vi "Update_FFID_Bkgnd_info.vi"(1 "Specific Bkgnd Meas?":bool, 2 "c^2 (ppm^2)":dbl[](array[numeric]), 3 "C (ppm)":dbl[](array[numeric])) -> ()   [LabVIEW 2010]
uses:
  Globals/Meas_global.vi
  Globals/Plug_in_data_global.vi
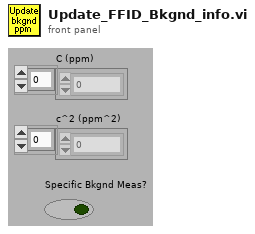
[diagram p1: front panel]
types:
  T1 = typedef "Analysis_info_cluster.ctl" = cluster{"Colour":u32, "Inst type":T2, "Inst name":string, "Symbol":string, "Code name":string, "Extra Info":string, "Inst Array":T3, "Index":i32, "Voltage Index":i32, "Extra Titles":string[], "Extra Values":string[]}
  T2 = typedef "Inst_type.ctl" = enum16{"Propeller anemometer", "Raw voltage", "Pressure Transducer", "Pitot-static tube", "Preston tube", "Hot wire", "Cross wire 1", "Cross wire 2", "Generic Linear", "Generic Polynomial", "Generic BackPoly", "Fast FID", "Thermocouple", "Cold wire", "Pulsed Wire", "LDA Vel", "LDA Tran time", "LDA Arr time"}
  T3 = typedef "Instrument_Array.ctl" = enum16{"PWA", "LDA", "Analogue"}
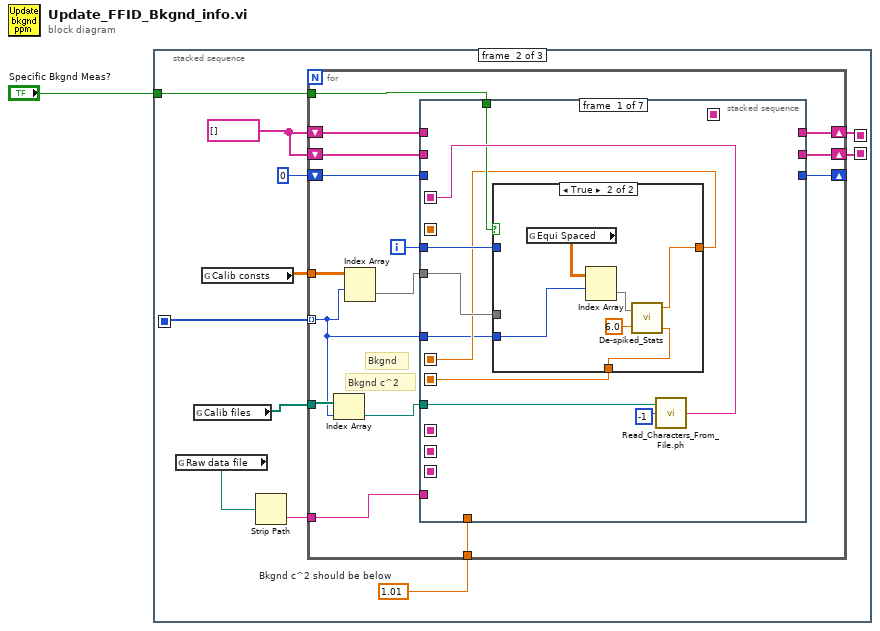
[diagram p0: block diagram]
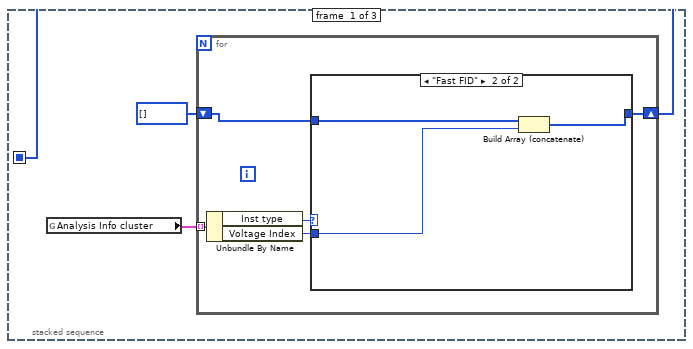
[diagram p2: hidden frame]
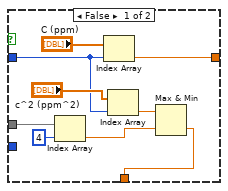
[diagram p4: hidden frame]
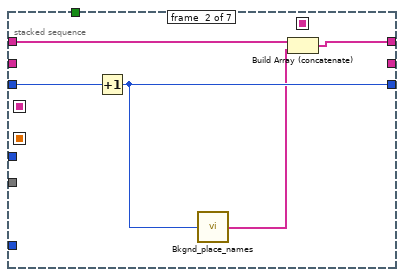
[diagram p5: hidden frame]
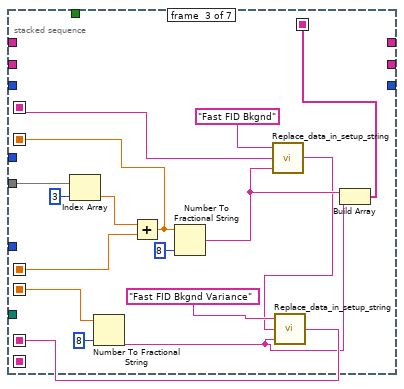
[diagram p6: hidden frame]
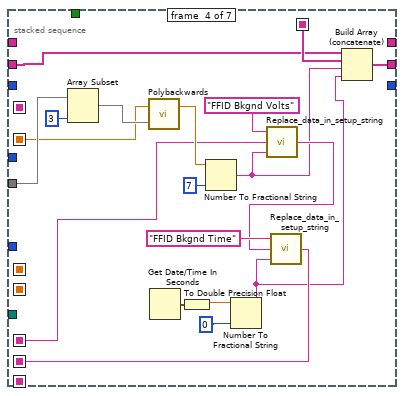
[diagram p7: hidden frame]
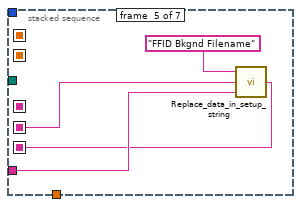
[diagram p8: hidden frame]
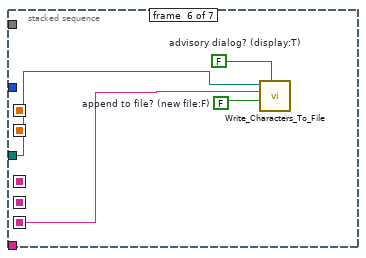
[diagram p9: hidden frame]
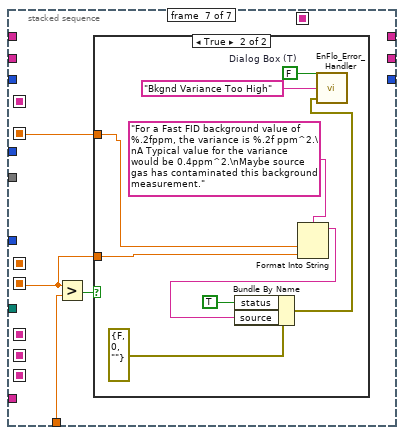
[diagram p10: hidden frame]
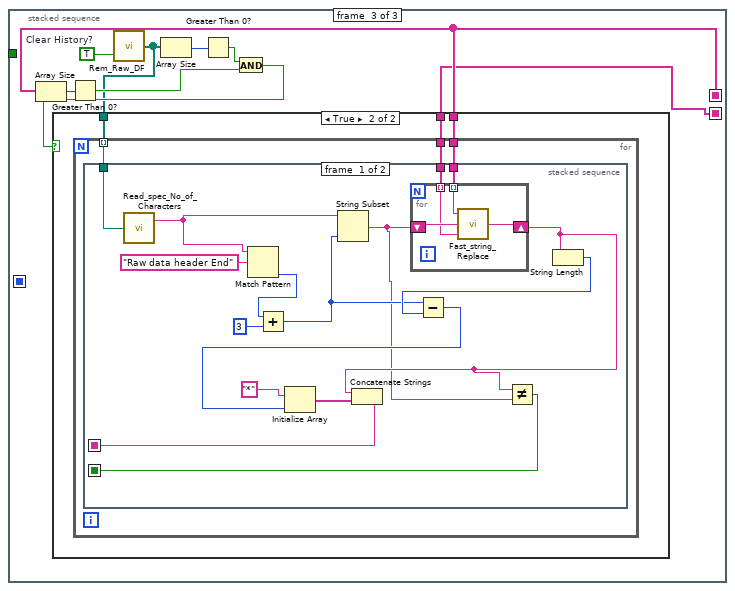
[diagram p12: hidden frame]
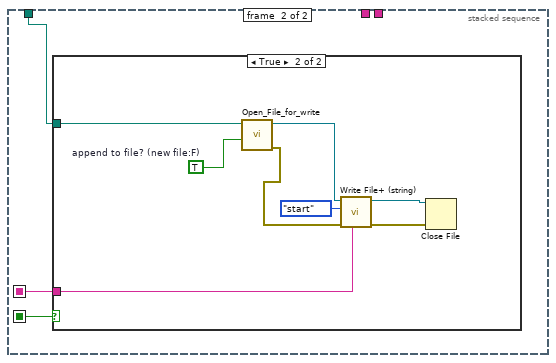
[diagram p14: hidden frame]
diagram:
  n1 = stacked-sequence {
    seq-local: [_ w18 _] -> [_ _ w127]
    seq-local: [_ w17 _] -> [_ _ w126]
    seq-local: [w2 _ _] -> [_ w15 _]
    tunnel: "Specific Bkgnd Meas?" -> [_ w14 _]
    frame #0 {
      n2 = global read "Meas_global.vi" "Analysis Info cluster"() -> (w3:T1[])
      n3 = for {
        shift-right: [w6] -> w2
        shift-left: i32[] [] -> [w8]
        tunnel: w3 -> [w5] mode=indexing
        n4 = Unbundle By Name(w5) -> ("Inst type"=w9:T2, "Voltage Index"=w7:i32)
        n5 = case shown="\"Fast FID\"" w9 {
          tunnel: w8 -> [w10 w13]
          tunnel: w7 -> [_ w12]
          tunnel: [w10 w11] -> w6
          frame "Propeller anemometer", Default {
          }
          frame "Fast FID" {
            n6 = Build Array (concatenate)(w13, w12) -> (w11:i32[])
          }
        }
      }
    }
    frame #1 {
      w16 = 1.01  # Bkgnd c^2 should be below
      w19 = string[] []
      n7 = global read "Meas_global.vi" "Raw data file"() -> (w22:path)
      n8 = global read "Meas_global.vi" "Calib files"() -> (w23:path[])
      n9 = global read "Meas_global.vi" "Calib consts"() -> (w24:dbl[][])
      n10 = Strip Path(path=w22) -> (name=w21:string)  [unwired: 1 out]
      n11 = for {
        tunnel: w24 -> [w31]
        tunnel: w23 -> [w30]
        tunnel: w21 -> [w39]
        shift-right: [w37] -> _
        shift-left: 0 -> [w38]
        shift-right: [w33] -> w17
        shift-left: w19 -> [w34]
        shift-right: [w35] -> w18
        shift-left: w19 -> [w36]
        tunnel: w16 -> [w32]
        tunnel: w15 -> [w25] mode=indexing
        tunnel: w14 -> [w27]
        i -> [w26]
        # "Bkgnd c^2"
        # "Bkgnd"
        n12 = Index Array(array=w30, index=w25) -> (element=w29:path)
        n13 = Index Array(array=w31, index (row)=w25) -> (element=w28:dbl[])  [unwired: 1 in]
        n14 = stacked-sequence {
          seq-local: [w47 _ _ _ _ _ _] -> [_ _ w79 _ _ _ _]
          seq-local: [_ _ w77 _ _ _ _] -> [_ _ _ w92 _ _ _]
          seq-local: [_ _ w75 _ _ _ _] -> [_ _ _ w100 _ _ w115]
          seq-local: [_ _ _ w90 _ _ _] -> [_ _ _ _ w104 _ _]
          seq-local: [_ _ _ _ w105 _ _] -> [_ _ _ _ _ w109 _]
          seq-local: [_ _ w71 _ _ _ _] -> [_ _ _ w89 _ _ _]
          seq-local: [w44 _ _ _ _ _ _] -> [_ _ w70 _ _ _ w114]
          seq-local: [w41 _ _ _ _ _ _] -> [_ _ w69 _ _ _ _]
          tunnel: w28 -> [w43 _ w84 w103 _ _ _]
          tunnel: w29 -> [w46 _ _ _ _ w108 _]
          tunnel: w39 -> [_ _ _ _ w106 _ _]
          tunnel: w38 -> [_ w68 _ _ _ _ _]
          tunnel: [_ w67 _ _ _ _ _] -> w37
          tunnel: w36 -> [_ w65 _ _ _ _ _]
          tunnel: [_ w64 _ _ _ _ _] -> w35
          tunnel: w34 -> [_ _ _ w86 _ _ _]
          tunnel: [_ _ _ w85 _ _ _] -> w33
          tunnel: w32 -> [_ _ _ _ _ _ w112]
          tunnel: w27 -> [w45 _ _ _ _ _ _]
          tunnel: w26 -> [w42 _ _ _ _ _ _]
          tunnel: w25 -> [w40 _ _ _ _ _ _]
          frame #0 {
            n15 = case shown="True" w45 {
              tunnel: [w49 w58] -> w44
              tunnel: w43 -> [w57 _]
              tunnel: w42 -> [w52 _]
              tunnel: [w54 w59] -> w41
              tunnel: w40 -> [_ w62]
              frame False {
                n16 = Index Array(array=w57, index=4) -> (element=w50:dbl)
                n17 = Index Array(array="C (ppm)", index=w52) -> (element=w54:dbl)
                n18 = Index Array(array="c^2 (ppm^2)", index=w52) -> (element=w51:dbl)
                n19 = Max & Min(x=w51, y=w50) -> (min(x,y)=w49:dbl)  [unwired: 1 out]
              }
              frame True {
                n20 = global read "Plug_in_data_global.vi" "Equi Spaced"() -> (w63:dbl[][])
                n21 = Index Array(array=w63, index (row)=w62) -> (element=w60:dbl[])  [unwired: 1 in]
                n22 = call "De-spiked_Stats.vi"("Raw Signal"=w60, "No of st dev to chop at"=6.0) -> ("mean"=w59:dbl, "variance"=w58:dbl)  [unwired: 1 out]
              }
            }
            n23 = call "Read_Characters_From_File.ph.vi"("file path (dialog if empty)"=w46, "number of characters (all:-1)"=-1) -> ("character string"=w47:string)  [unwired: 7 out]
          }
          frame #1 {
            n24 = Increment(x=w68) -> (x+1=w67:i32)
            n25 = call "Bkgnd_place_names.vi"("Numeric"=w67) -> ("Array"=w66:string[])
            n26 = Build Array (concatenate)(w65, w66) -> (w64:string[])
          }
          frame #2 {
            n27 = Index Array(array=w84, index=3 ("Index")) -> (element=w82:dbl)
            n28 = Number To Fractional String(number=w70, precision (6)=i16 8) -> (F-format string=w72:string)  [unwired: 2 out]
            n29 = Add(x=w82, y=w69) -> (x+y=w75:dbl)
            n30 = Number To Fractional String(number=w75, precision (6)=i16 8) -> (F-format string=w74:string)  [unwired: 2 out]
            n31 = call "Replace_data_in_setup_string.vi"("New data string"=w74, "Input string"=w79, "Variable name"="Fast FID Bkgnd") -> ("Appended string"=w73:string)
            n32 = call "Replace_data_in_setup_string.vi"("New data string"=w72, "Input string"=w73, "Variable name"="Fast FID Bkgnd Variance") -> ("Appended string"=w77:string)
            n33 = Build Array(w74, w72) -> (w71:string[])
          }
          frame #3 {
            n34 = Array Subset(array=w103, length=3 ("index")) -> (w101:dbl[])  [unwired: 1 in]
            n35 = call "Polybackwards.vi"("Coefficients"=w101, "Y input"=w100) -> ("X output"=w99:dbl)  [unwired: 1 out]
            n36 = Get Date/Time In Seconds() -> (seconds since 1Jan1904=w96:timestamp)
            n37 = To Double Precision Float(number=w96) -> (double precision float=w94:dbl)
            n38 = Number To Fractional String(number=w99, precision (6)=i16 7) -> (F-format string=w88:string)  [unwired: 2 out]
            n39 = Number To Fractional String(number=w94, precision (6)=i16 0) -> (F-format string=w87:string)  [unwired: 2 out]
            n40 = call "Replace_data_in_setup_string.vi"("New data string"=w88, "Input string"=w92, "Variable name"="FFID Bkgnd Volts") -> ("Appended string"=w91:string)
            n41 = call "Replace_data_in_setup_string.vi"("New data string"=w87, "Input string"=w91, "Variable name"="FFID Bkgnd Time") -> ("Appended string"=w90:string)
            n42 = Build Array (concatenate)(w86, w89, w88, w87) -> (w85:string[])
          }
          frame #4 {
            n43 = call "Replace_data_in_setup_string.vi"("New data string"=w106, "Input string"=w104, "Variable name"="FFID Bkgnd Filename") -> ("Appended string"=w105:string)
          }
          frame #5 {
            w110 = FALSE  # advisory dialog? (display:T)
            w111 = FALSE  # append to file? (new file:F)
            n44 = call "Write_Characters_To_File.vi"("file path (dialog if empty)"=w108, "advisory dialog? (display:T)"=w110, "character string"=w109, "append to file? (new file:F)"=w111) -> ()  [unwired: 1 in, 4 out]
          }
          frame #6 {
            n45 = Greater?(x=w114, y=w112) -> (0:w113:bool)
            n46 = case shown="True" w113 {
              tunnel: w114 -> [_ w121]
              tunnel: w115 -> [_ w120]
              frame False {
              }
              frame True {
                w116 = FALSE  # Dialog Box (T)
                n47 = Format Into String(format string="For a Fast FID background value of %.2fppm, the variance is %.2f ppm^2.\nA Typical value for the variance would be 0.4ppm^2.\nMaybe source gas has contaminated this background measurement.", w120, w121) -> (resulting string=w118:string)  [unwired: 2 in, 1 out]
                n48 = Bundle By Name(cluster=errorcluster {"status"=FALSE, "code"=0, "source"=""} ("error in (no error)"), "status"=TRUE, "source"=w118) -> (w117:errorcluster)
                n49 = call "EnFlo_Error_Handler.vi"("error in (no error)"=w117, "Error Type"="Bkgnd Variance Too High", "Dialog Box (T)"=w116) -> ()  [unwired: 3 out]
              }
            }
          }
        }
      }
    }
    frame #2 {
      w125 = TRUE  # Clear History?
      n50 = Array Size(array=w127) -> (size(s)=w132:i32)
      n51 = Greater Than 0?(x=w132) -> (x > 0?=w130:bool)
      n52 = call "Rem_Raw_DF.vi"("Clear History?"=w125) -> ("List of Filenames"=w128:path[])  [unwired: 1 in]
      n53 = Array Size(array=w128) -> (size(s)=w133:i32)
      n54 = Greater Than 0?(x=w133) -> (x > 0?=w131:bool)
      n55 = And(x=w131, y=w130) -> (x .and. y?=w129:bool)
      n56 = case shown="True" w129 {
        tunnel: w128 -> [_ w136]
        tunnel: w127 -> [_ w135]
        tunnel: w126 -> [_ w134]
        frame False {
        }
        frame True {
          n57 = for {
            tunnel: w136 -> [w137] mode=indexing
            tunnel: w135 -> [w139]
            tunnel: w134 -> [w138]
            n58 = stacked-sequence {
              seq-local: [w143 _] -> [_ w161]
              seq-local: [w141 _] -> [_ w160]
              tunnel: w139 -> [w151 _]
              tunnel: w138 -> [w150 _]
              tunnel: w137 -> [w144 w162]
              frame #0 {
                n59 = call "Read_spec_No_of_Characters.vi"("Filename"=w144) -> ("character string"=w152:string)  [unwired: 1 out]
                n60 = Match Pattern(string=w152, regular expression="Raw data header End") -> (offset past match=w154:i32)  [unwired: 4 out]
                n61 = Add(x=w154, y=3) -> (x+y=w148:i32)
                n62 = String Subset(string=w152, length (rest)=w148) -> (substring=w140:string)  [unwired: 1 out]
                n63 = for {
                  shift-right: [w158] -> w142
                  shift-left: w140 -> [w159]
                  tunnel: w151 -> [w157] mode=indexing
                  tunnel: w150 -> [w156] mode=indexing
                  n64 = call "Fast_string_Replace.vi"("Replace match with:"=w156, "Input String"=w159, "regular expression"=w157) -> ("Output String"=w158:string)  [unwired: 2 out]
                }
                n65 = Not Equal?(x=w142, y=w140) -> (x != y?=w141:bool)
                n66 = String Length(string=w142) -> (length=w149:i32)
                n67 = Subtract(x=w148, y=w149) -> (x-y=w146:i32)
                n68 = Initialize Array("*", w146) -> (w145:string[])
                n69 = Concatenate Strings(w142, w145) -> (w143:string)
              }
              frame #1 {
                n70 = case shown="True" w160 {
                  tunnel: w162 -> [_ w170]
                  tunnel: w161 -> [_ w163]
                  frame False {
                  }
                  frame True {
                    w169 = TRUE  # append to file? (new file:F)
                    n71 = call "Open_File_for_write.vi"("append to file? (new file:F)"=w169, "file path"=w170) -> ("error out"=w166:errorcluster, "refnum"=w167:refnum<file>)  [unwired: 1 in, 7 out]
                    n72 = call <vilib>:"Write File+ (string).vi"("string"=w163, "error in (no error)"=w166, "pos mode (rel. to end:1)"=enum16{"start", "end", "current"}."start", "refnum"=w167) -> ("error out"=w164:errorcluster, "dup refnum"=w165:refnum<file>)  [unwired: 1 in, 3 out]
                    n73 = Close File(refnum=w165, error in=w164) -> ()  [unwired: 2 out]
                  }
                }
              }
            }
          }
        }
      }
    }
  }
